vi "ma_sml_Advanced Spectrum Peak Search.vi"(4 "peaks near frequencies":T1={"Frequencies"=[], "Tolerance (Hz)"=100.0} {"Tolerance (Hz)" format="%_4p"; "Frequencies" format="%_4p"}, 6 "highest n peaks":i32=1, 7 "threshold":dbl format="%.2f", 8 "error in (no error)":errorcluster, 9 "peak search mode":u16(ring) items=["Threshold", "Highest N Peaks", "Peaks Near Frequencies"], 10 "spectral info":T3 {"window" items=["Rectangle"=0, "Hanning"=1, "Hamming"=2, "Blackman-Harris"=3, "Exact Blackman"=4, "Blackman"=5, "Flat Top"=6, "4 Term B-Harris "=7, "7 Term B-Harris"=8, "Low Sidelobe"=9, "Blackman Nuttall"=11, "Triangle"=30, "Bartlett-Hanning"=31, "Bohman"=32, "Parzen"=33, "Welch"=34, "Kaiser"=60, "Dolph-Chebyshev"=61, "Gaussian"=62]}, 11 "spectrum":T2={"f0"=1.0, "df"=1.0, "spectrum"=[]} {"spectrum" format="%.2f"; "df" format="%.2f"; "f0" format="%.2f"}) -> (0 "error out":errorcluster, 2 "# of peaks":i32, 3 "peaks":cluster{"frequency":dbl, "Value":dbl}[](array[cluster]) {"Value" format="%.2f"; "frequency" format="%.2f"})   [LabVIEW 2020, in "NI_MAPro.lvlib"]
uses:
  NI_MAPro.lvlib
  ma_sml_Spectral Info.ctl
  ma_sml_Spectrum Cluster (real).ctl
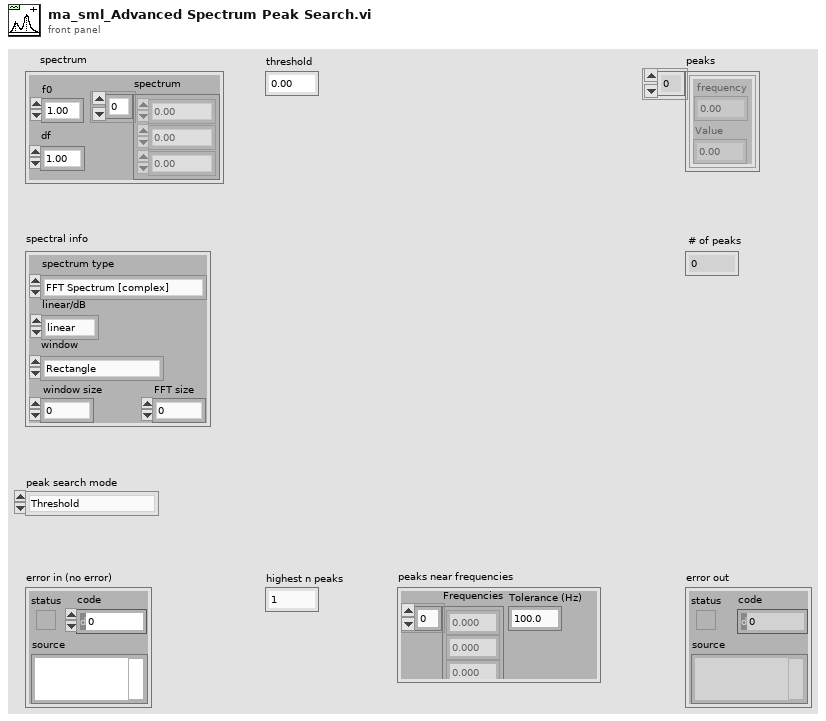
[diagram p1: front panel]
types:
  T1 = cluster{"Frequencies":dbl[], "Tolerance (Hz)":dbl}
  T2 = typedef "NI_MAPro.lvlib/ma_sml_Spectrum Cluster (real).ctl" = cluster{"f0":dbl, "df":dbl, "spectrum":dbl[]}
  T3 = typedef "NI_MAPro.lvlib/ma_sml_Spectral Info.ctl" = cluster{"spectrum type":enum16{"FFT Spectrum [complex]", "Amplitude [Magnitude]", "Power [Magnitude^2]", "Cross Spectrum [complex]", "Frequency Response [Complex]"}, "linear/dB":enum16{"linear", "dB"}, "window":u16, "window size":i32, "FFT size":i32}
  T4 = enum16{"FFT Spectrum [complex]", "Amplitude [Magnitude]", "Power [Magnitude^2]", "Cross Spectrum [complex]", "Frequency Response [Complex]"}
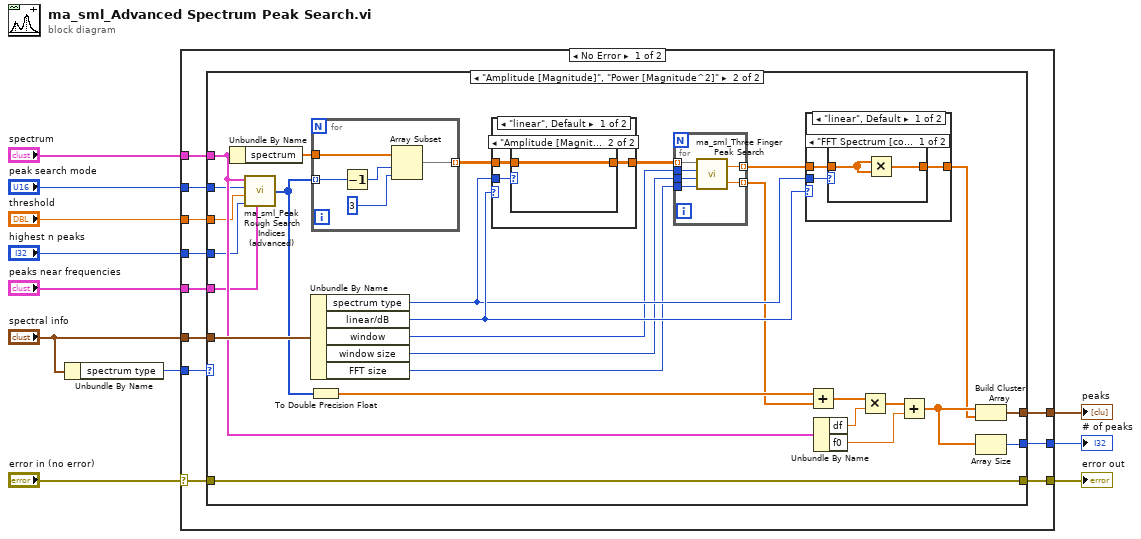
[diagram p0: block diagram]
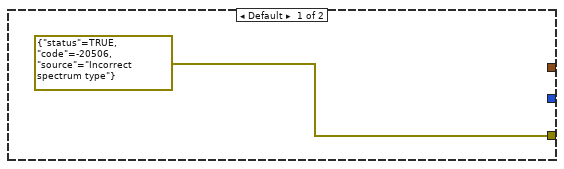
[diagram p2: hidden frame]
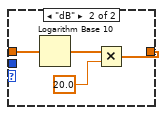
[diagram p4: hidden frame]
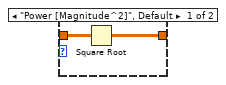
[diagram p5: hidden frame]
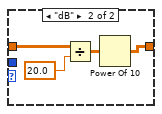
[diagram p6: hidden frame]
diagram:
  n1 = Unbundle By Name("spectral info") -> ("spectrum type"=w8:T4)
  n2 = case shown="No Error" "error in (no error)" {
    selector: "error in (no error)" -> [w20 w82]
    tunnel: "spectral info" -> [w22 _]
    tunnel: [w19 w82] -> w10
    tunnel: w8 -> [w21 _]
    tunnel: [w18 _] -> w7
    tunnel: [w17 _] -> w6
    tunnel: "spectrum" -> [w16 _]
    tunnel: "peak search mode" -> [w15 _]
    tunnel: "threshold" -> [w14 _]
    tunnel: "highest n peaks" -> [w13 _]
    tunnel: "peaks near frequencies" -> [w12 _]
    frame No Error {
      n3 = case shown="\"Amplitude [Magnitude]\", \"Power [Magnitude^2]\"" w21 {
        tunnel: w22 -> [_ w38]
        tunnel: w20 -> [_ w34]
        tunnel: [errorcluster {"status"=TRUE, "code"=-20506, "source"="Incorrect spectrum type"} ("error IO") w34] -> w19
        tunnel: [_ w33] -> w18
        tunnel: [_ w32] -> w17
        tunnel: w16 -> [_ w29]
        tunnel: w15 -> [_ w27]
        tunnel: w14 -> [_ w26]
        tunnel: w13 -> [_ w25]
        tunnel: w12 -> [_ w24]
        frame Default {
        }
        frame "Amplitude [Magnitude]", "Power [Magnitude^2]" {
          n4 = Unbundle By Name(w29) -> ("spectrum"=w40:dbl[])
          n5 = call "ma_sml_Peak Rough Search Indices (advanced).vi"("spectrum"=w29, "peak search mode"=w27, "threshold"=w26, "highest n peaks"=w25, "peaks near frequencies"=w24) -> ("peak indices"=w28:i32[])
          n6 = Unbundle By Name(w38) -> ("spectrum type"=w43:T4, "linear/dB"=w44:enum16{"linear", "dB"}, "window"=w39:u16, "window size"=w42:i32, "FFT size"=w41:i32)
          n7 = To Double Precision Float(number=w28) -> (double precision float=w35:dbl[])
          n8 = for {
            tunnel: w28 -> [w77] mode=indexing
            tunnel: w40 -> [w81]
            tunnel: [w78] -> w47 mode=indexing
            n9 = Decrement(x=w77) -> (x-1=w79:i32)
            n10 = Array Subset(array=w81, index=w79, length=3 ("Array Length")) -> (w78:dbl[])
          }
          n11 = case shown="\"linear\", Default" w44 {
            tunnel: w47 -> [w69 w76]
            tunnel: [w68 w75] -> w46
            tunnel: w43 -> [w67 _]
            frame "linear", Default {
              n12 = case shown="\"Amplitude [Magnitude]\"" w67 {
                tunnel: w69 -> [w71 w72]
                tunnel: [w70 w72] -> w68
                frame "Power [Magnitude^2]", Default {
                  n13 = Square Root(x=w71) -> (sqrt(x)=w70:dbl[][])
                }
                frame "Amplitude [Magnitude]" {
                }
              }
            }
            frame "dB" {
              n14 = Divide(x=w76, y=20.0 ("x")) -> (x/y=w73:dbl[][])
              n15 = Power Of 10(x=w73) -> (10^x=w75:dbl[][])
            }
          }
          n16 = for {
            tunnel: [w66] -> w31 mode=indexing
            tunnel: [w65] -> w30 mode=indexing
            tunnel: w46 -> [w64] mode=indexing
            tunnel: w39 -> [w63]
            tunnel: w42 -> [w62]
            tunnel: w41 -> [w61]
            n17 = call "ma_sml_Three Finger Peak Search.vi"("FFT Size"=w61, "window length"=w62, "window"=w63, "three fingers"=w64) -> ("freq"=w65:dbl, "amplitude"=w66:dbl)
          }
          n18 = case shown="\"linear\", Default" w44 {
            tunnel: w31 -> [w53 w60]
            tunnel: [w52 w59] -> w36
            tunnel: w43 -> [w51 _]
            frame "linear", Default {
              n19 = case shown="\"FFT Spectrum [complex]\", Default" w51 {
                tunnel: w53 -> [w54 w56]
                tunnel: [w55 w56] -> w52
                frame "FFT Spectrum [complex]", Default {
                  n20 = Multiply(x=w54, y=w54) -> (x*y=w55:dbl[])
                }
                frame "Amplitude [Magnitude]" {
                }
              }
            }
            frame "dB" {
              n21 = Logarithm Base 10(1:w60) -> (0:w58:dbl[])
              n22 = Multiply(x=w58, y=20.0) -> (x*y=w59:dbl[])
            }
          }
          n23 = Add(x=w35, y=w30) -> (x+y=w45:dbl[])
          n24 = Unbundle By Name(w29) -> ("df"=w49:dbl, "f0"=w48:dbl)
          n25 = Multiply(x=w45, y=w49) -> (x*y=w50:dbl[])
          n26 = Add(x=w50, y=w48) -> (x+y=w37:dbl[])
          n27 = Build Cluster Array(w37, w36) -> (w33:cluster{dbl, "amplitude":dbl}[])
          n28 = Array Size(array=w37) -> (size(s)=w32:i32)
        }
      }
    }
    frame Error {
    }
  }
  "error out" <- w10
  "peaks" <- w7
  "# of peaks" <- w6
